vi "SubVI_Convolution_Build Kenel #.vi"(1 "Kernel Size":i32=3 min=3 max=201 step=2) -> (0 "Kernel":sgl[][](array[numeric]))   [LabVIEW 2013]
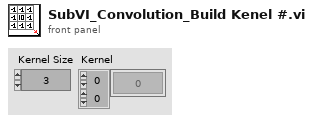
[diagram p1: front panel]
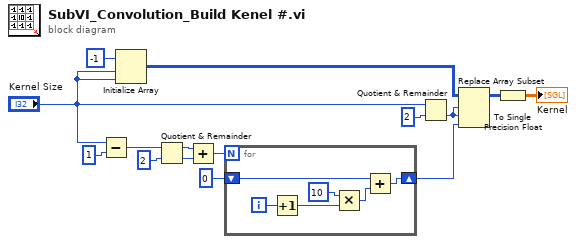
[diagram p0: block diagram]
diagram:
  n1 = Subtract(x="Kernel Size", y=1) -> (x-y=w10:i32)
  n2 = Initialize Array(-1 ("element"), "Kernel Size", "Kernel Size") -> (w15:i32[][])
  n3 = Quotient & Remainder(x=w10, y=2) -> (x-y*floor(x/y)=w6:i32, floor(x/y)=w5:i32)
  n4 = Add(x=w6, y=w5) -> (x+y=w4:i32)
  n5 = for {
    N: w4 -> [_]
    shift-right: [w19] -> w3
    shift-left: 0 -> [w18]
    i -> [w17]
    n6 = Increment(x=w17) -> (x+1=w16:i32)
    n7 = Multiply(x=10, y=w16) -> (x*y=w20:i32)
    n8 = Add(x=w18, y=w20) -> (x+y=w19:i32)
  }
  n9 = Quotient & Remainder(x="Kernel Size", y=2) -> (floor(x/y)=w13:i32)  [unwired: 1 out]
  n10 = Replace Array Subset(array=w15, new element=w3, index (row)=w13, index (col)=w13) -> (w2:i32[][])
  n11 = To Single Precision Float(number=w2) -> (single precision float=→"Kernel":sgl[][])
